vi "Default.vi"(8 "error in (no error)":errorcluster, 11 "Channel in":refnum<class "Channel.lvclass">) -> (0 "error out":errorcluster, 2 "Default":string, 3 "Channel out":refnum<class "Channel.lvclass">)   [LabVIEW 2020, in "VolatusConfig.lvlib" / "Channel.lvclass"]
uses:
  Channel.lvclass
  Channel.lvclass/Channel.ctl
  lv-cdm/CDM-Config/Config Element/Config Element.lvclass
  VolatusConfigElement/VolatusConfigElement.lvclass
  C:/dev/lv20CE/relink/lv-volatus/VolatusConfig/VolatusConfigElement/VolatusConfigElement.lvclass
  C:/dev/lv20CE/relink/lv-volatus/VolatusConfig/Channel/Channel.lvclass
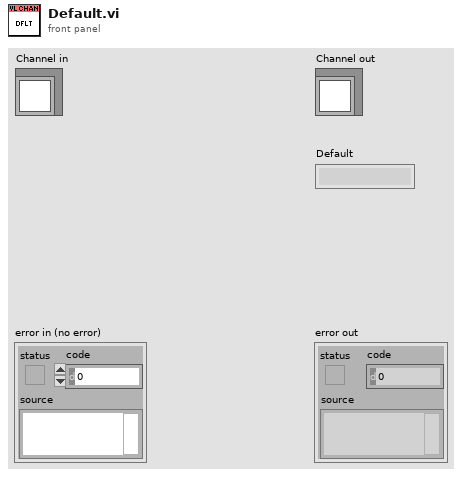
[diagram p1: front panel]
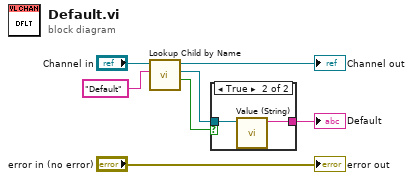
[diagram p0: block diagram]
diagram:
  n1 = call "Lookup Child by Name.vi"("Child Name"="Default" ("Name"), "VolatusConfigElement in"="Channel in") -> ("Found"=w3:bool, "Child"=w2:refnum<class "Config Element.lvclass">, "VolatusConfigElement out"=→"Channel out":refnum<class "Channel.lvclass">)  [unwired: 6 in, 1 out]
  n2 = case shown="True" w3 {
    tunnel: w2 -> [_ w9]
    tunnel: [_ w8] -> w5
    frame False {
    }
    frame True {
      n3 = call "Value (String).vi"("Config Element in"=w9) -> ("String Value"=w8:string)  [unwired: 9 in, 1 out]
    }
  }
  "Default" <- w5
  "error out" <- "error in (no error)"
